vi "sprezyna-masny.vi"(1 "n":i32=3 min=3 max=8, 3 "w":dbl=20.0 min=20.0 max=50.0, 4 "h":dbl, 5 "x0y0":cluster{dbl, dbl}, 6 "Pic in":picture) -> (0 "Pic out":picture)   [LabVIEW 2019]
panel:
  in  "y":dbl=10.0 min=10.0
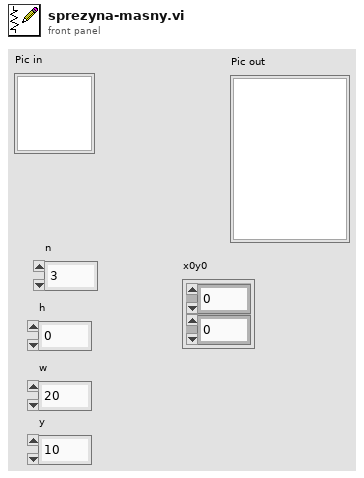
[diagram p1: front panel]
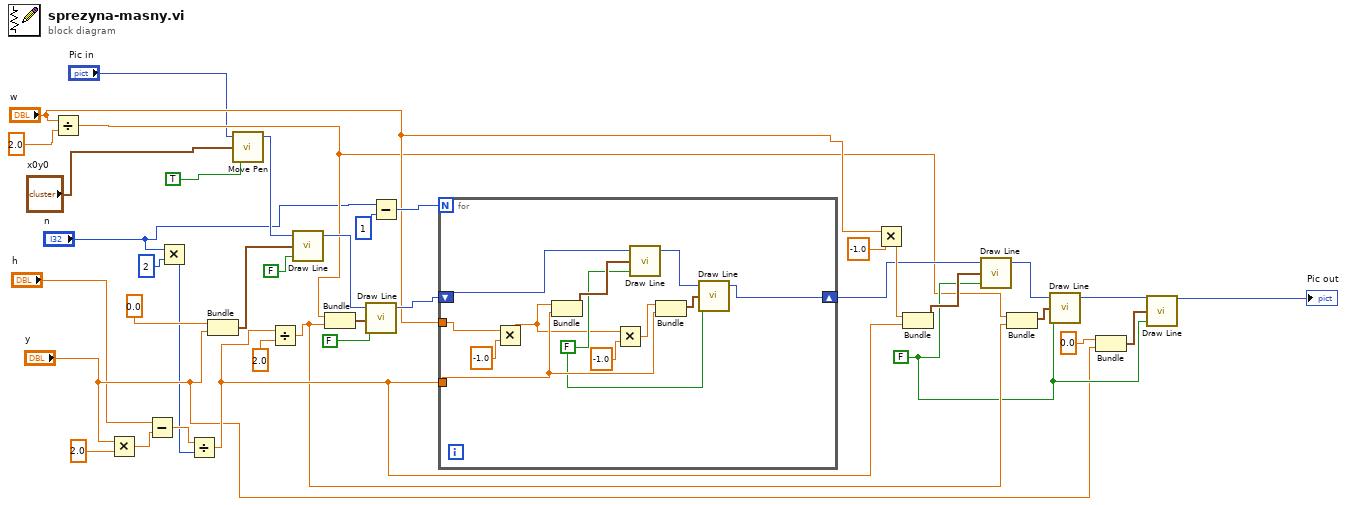
[diagram p0: block diagram]
diagram:
  w12 = FALSE ("absolute coordinates?(T)")
  n1 = Divide(x="w", y=2.0) -> (x/y=w8:dbl)
  n2 = Multiply(x="y", y=2.0) -> (x*y=w38:dbl)
  n3 = Subtract(x="h", y=w38) -> (x-y=w36:dbl)
  n4 = Multiply(x="n", y=2) -> (x*y=w3:i32)
  n5 = Divide(x=w36, y=w3) -> (x/y=w16:dbl)
  n6 = Bundle("element"=0.0, "y"="y") -> (w34:cluster{"element":dbl, "y":dbl})  [unwired: 1 in]
  n7 = call <vilib>:"Move Pen.vi"("absolute coordinates?(T)"=TRUE, "new position"="x0y0", "picture"="Pic in") -> ("new picture"=w31:picture)  [unwired: 2 in]
  n8 = Divide(x=w16, y=2.0) -> (x/y=w15:dbl)
  n9 = call <vilib>:"Draw Line.vi"("picture"=w31, "end point"=w34, "absolute coordinates?(T)"=FALSE) -> ("new picture"=w28:picture)  [unwired: 6 in]
  n10 = Bundle(w8, w15) -> (w25:cluster{dbl, dbl})  [unwired: 1 in]
  n11 = call <vilib>:"Draw Line.vi"("picture"=w28, "end point"=w25, "absolute coordinates?(T)"=FALSE) -> ("new picture"=w26:picture)  [unwired: 6 in]
  n12 = Subtract(x="n", y=1) -> (x-y=w23:i32)
  n13 = for {
    N: w23 -> [_]
    shift-right: [w42] -> w14
    shift-left: w26 -> [w50]
    tunnel: w16 -> [w47]
    tunnel: "w" -> [w40]
    w43 = FALSE ("absolute coordinates?(T)")
    n14 = Multiply(x=w40, y=-1.0) -> (x*y=w39:dbl)
    n15 = Bundle(w39, w47) -> (w49:cluster{dbl, dbl})  [unwired: 1 in]
    n16 = Multiply(x=w39, y=-1.0) -> (x*y=w45:dbl)
    n17 = call <vilib>:"Draw Line.vi"("picture"=w50, "end point"=w49, "absolute coordinates?(T)"=w43) -> ("new picture"=w48:picture)  [unwired: 6 in]
    n18 = Bundle(w45, w47) -> (w44:cluster{dbl, dbl})  [unwired: 1 in]
    n19 = call <vilib>:"Draw Line.vi"("picture"=w48, "end point"=w44, "absolute coordinates?(T)"=w43) -> ("new picture"=w42:picture)  [unwired: 6 in]
  }
  n20 = Multiply(x="w", y=-1.0) -> (x*y=w17:dbl)
  n21 = Bundle(w17, w16) -> (w19:cluster{dbl, dbl})  [unwired: 1 in]
  n22 = call <vilib>:"Draw Line.vi"("picture"=w14, "end point"=w19, "absolute coordinates?(T)"=w12) -> ("new picture"=w20:picture)  [unwired: 6 in]
  n23 = Bundle(w8, w15) -> (w22:cluster{dbl, dbl})  [unwired: 1 in]
  n24 = call <vilib>:"Draw Line.vi"("picture"=w20, "end point"=w22, "absolute coordinates?(T)"=w12) -> ("new picture"=w13:picture)  [unwired: 6 in]
  n25 = Bundle("element"=0.0, "y"="y") -> (w9:cluster{"element":dbl, "y":dbl})  [unwired: 1 in]
  n26 = call <vilib>:"Draw Line.vi"("picture"=w13, "end point"=w9, "absolute coordinates?(T)"=w12) -> ("new picture"=→"Pic out":picture)  [unwired: 6 in]
